vi "Disabled Test 0003.vi"(8 "error in (no error)":errorcluster) -> (0 "error out":errorcluster)   [LabVIEW 2013]
uses:
  classes/Assert/Assert.lvclass
  classes/Test/Test.lvclass
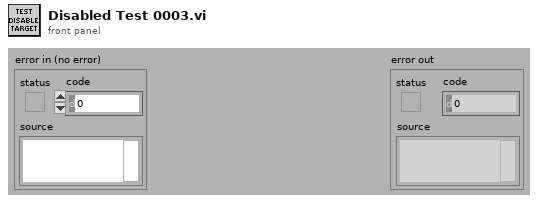
[diagram p1: front panel]
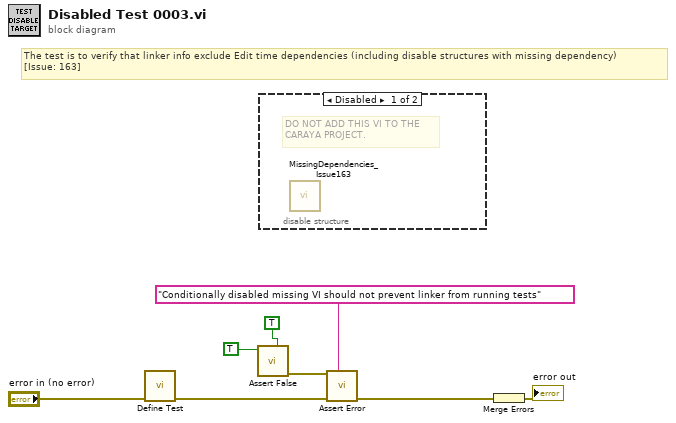
[diagram p0: block diagram]
diagram:
  # "The test is to verify that linker info exclude Edit time dependencies (including disable structures with missing dependency)\n[Issue: 163]"
  n1 = call "Define Test.vi"("error in (no error)"="error in (no error)") -> ("error out"=w1:errorcluster)  [unwired: 9 in, 1 out]
  n2 = call "Assert False.vi"("Assert Only? (F)"=TRUE, "False?"=TRUE ("True?")) -> ("error out"=w7:errorcluster)  [unwired: 8 in, 1 out]
  n3 = disable-structure shown="Disabled" {
    frame Disabled {
      # "DO NOT ADD THIS VI TO THE\nCARAYA PROJECT."
      n4 = call "MissingDependencies_Issue163.vi"() -> ()  [unwired: 12 in]
    }
    frame Enabled {
    }
  }
  n5 = call "Assert Error.vi"("Label"="Conditionally disabled missing VI should not prevent linker from running tests", "error in (no error)"=w1, "Error?"=w7) -> ("error out"=w3:errorcluster)  [unwired: 7 in, 1 out]
  n6 = Merge Errors(w3) -> (→"error out":errorcluster)
